vi "Get Registration.vi"(11 "Hello World Event in":refnum<class "Hello World Event.lvclass">) -> (2 "Registration":refnum<event-registration>)   [LabVIEW 2021, in "Hello World Event.lvlib" / "Hello World Event.lvclass"]
uses:
  Hello World Event.lvclass
  <vilib>/Nathan Davis/jettl/jettl/Msg Strategy/Msg Strategy.lvclass
  Hello World Event.lvclass/Hello World Event.ctl
  <vilib>/Nathan Davis/jettl/jettl/Event/Event.lvclass
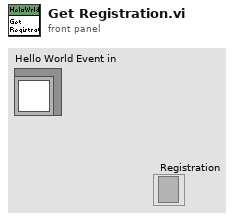
[diagram p1: front panel]
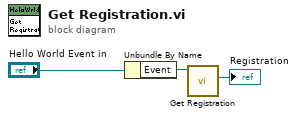
[diagram p0: block diagram]
diagram:
  n1 = Unbundle By Name("Hello World Event in") -> ("Event"=w2:refnum<class "Event.lvclass">)
  n2 = call-dynamic "Get Registration.vi"("Event in"=w2) -> ("Registration"=→"Registration":refnum<event-registration>)  [unwired: 10 in]
